vi "FPGA myRIOMain_v4.vi"() -> ()   [LabVIEW 2019]
doc: "Main FPGA VI\nUse the bitfile generated by this VI in the real-time code.\n\nFlip the channels for input and output"
uses:
  TypeDefs/AO mode TabCtrl.ctl
  TypeDefs/SamplingModeEnum.ctl
  <vilib>/rvi/Emulation/niFpgaGetClockAttributes.vi
  <vilib>/rvi/Emulation/niFpgaSctlEmulationGetInTimedLoop.vi
  <vilib>/rvi/Emulation/niFpgaEmulationReportErrorSimple.vi
  <vilib>/rvi/eio/common/nirviEmuTemplateMethod_errors.vi
  <vilib>/rvi/Emulation/niFpgaProcessEmulError.vi
  <vilib>/rvi/Emulation/niFpgaCriticalErrorInLSC.vi
  <vilib>/rvi/Emulation/niFpgaEmulationIsFPGAContextNoSignature.vi
  <vilib>/rvi/errors/niFpgaSetErrorForExecOnDevCompSimple.vi
  <vilib>/rvi/eio/common/nirviEmuReportErrorAndStop.vi
  <vilib>/rvi/DataTransferAndStorage/Container/Common/niFpgaContainerGetUniqueNameForEmu.vi
  <vilib>/rvi/FIFO/Fifo_Resource/nirvififoEmulationSetSize.vi
  <vilib>/rvi/FIFO/Fifo_Resource/nirviFifoEmulationQueueMgr.vi
  <instcachedir>/0/nirviFifoEmulationQueueMgr_E5CAEC123FF24DC58D834DCA3CDAA9B5.lvgen/nirviFifoEmulationQueueMgr_E5CAEC123FF24DC58D834DCA3CDAA9B5_003.vi
  <vilib>/Utility/error.llb/Clear Errors.vi
  <vilib>/rvi/FIFO/Fifo_Resource/nirvififoEmulationCreateLock.vi
  <vilib>/rvi/FIFO/Fifo_Resource/nirvififoEmulationObtainLock.vi
  <vilib>/rvi/FIFO/Fifo_Resource/nirvififoEmulationReleaseLock.vi
  <vilib>/rvi/occurrence/nirviWaitOnOccurrenceBase.vi
  <vilib>/rvi/errors/nirviReportUnexpectedCaseInternalError.vi
  <vilib>/rvi/errors/nirviReportUnexpectedCaseInternalError (U32).vi
  <vilib>/rvi/FIFO/Fifo_Resource/nirvififoEmulationDetermineInputValidOut.vi
  <vilib>/eio/EIONode/EIONode.xnode
  <vilib>/rvi/DataTransferAndStorage/Container/XNode/niFpgaContainer.xnode
  <vilib>/rvi/FIFO/Fifo_Resource/nirvififoEmulationRead.vi
  <vilib>/rvi/Analysis/measure/butterworth/XNode/niFpgaButterworthFilter.xnode
  <vilib>/rvi/FXPMathLib/FxpMul/XNode/nifxpmath_Multiplier.xnode
  <vilib>/rvi/FIFO/Fifo_Resource/nirvififoEmulationWrite.vi
  FPGA functions/FPGA functions.lvlib
  <vilib>/rvi/FXPMathLib/sim/FxpSim.dll
panel:
  in  "AI Process Time [ticks]":u32=120
  out "Sample Freq. \ntoo high?":bool
  out "Processing Loop time [ticks]":u32
  out "AI Process. Freq.\ntoo high?":bool
  in  "Scaled Butterworth Coeffs":i32[](array[numeric])=[-1036986264, 2110353124, 93741, -1058362983, 2131726043, 94691]
  in  "Sampling Mode":T1
  in  "Bit-resolution":i8=12
  in  "AO mode":T2
  in  "AO Out [V]":fxp<+/-,18,5> format="%#.6g"
  in  "AO enable?":bool
  out "AI In [V]":fxp<+/-,25,5> format="%#.6g"
  out "FPGA AO DMA\nOverflow?":bool
  out "Int. Output":i16
  out "Raw Int. Input":i16
  in  "Sample Time [ticks]":u32=120
  out "AO Loop time [ticks]":u32
  out "AI Loop time [ticks]":u32
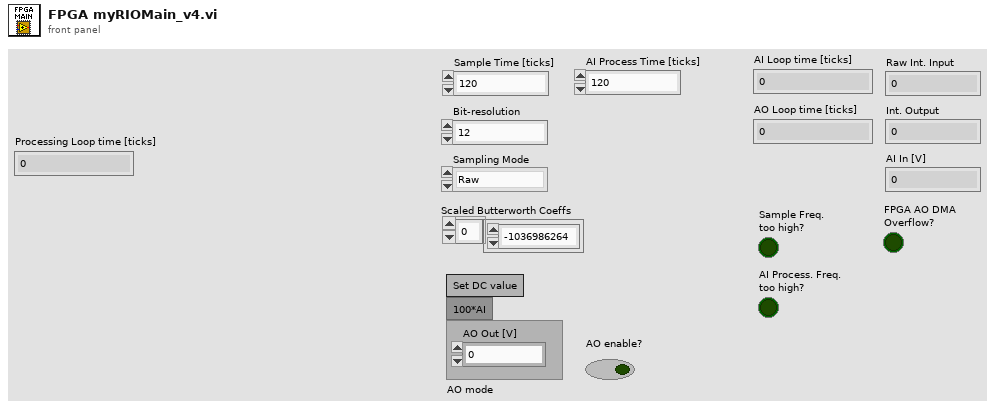
[diagram p1: front panel]
types:
  T1 = typedef "SamplingModeEnum.ctl" = enum16{"Raw", "LPF", "4 pt. Avg. + LPF"}
  T2 = typedef "AO mode TabCtrl.ctl" = enum32{"Set DC value", "100*AI"}
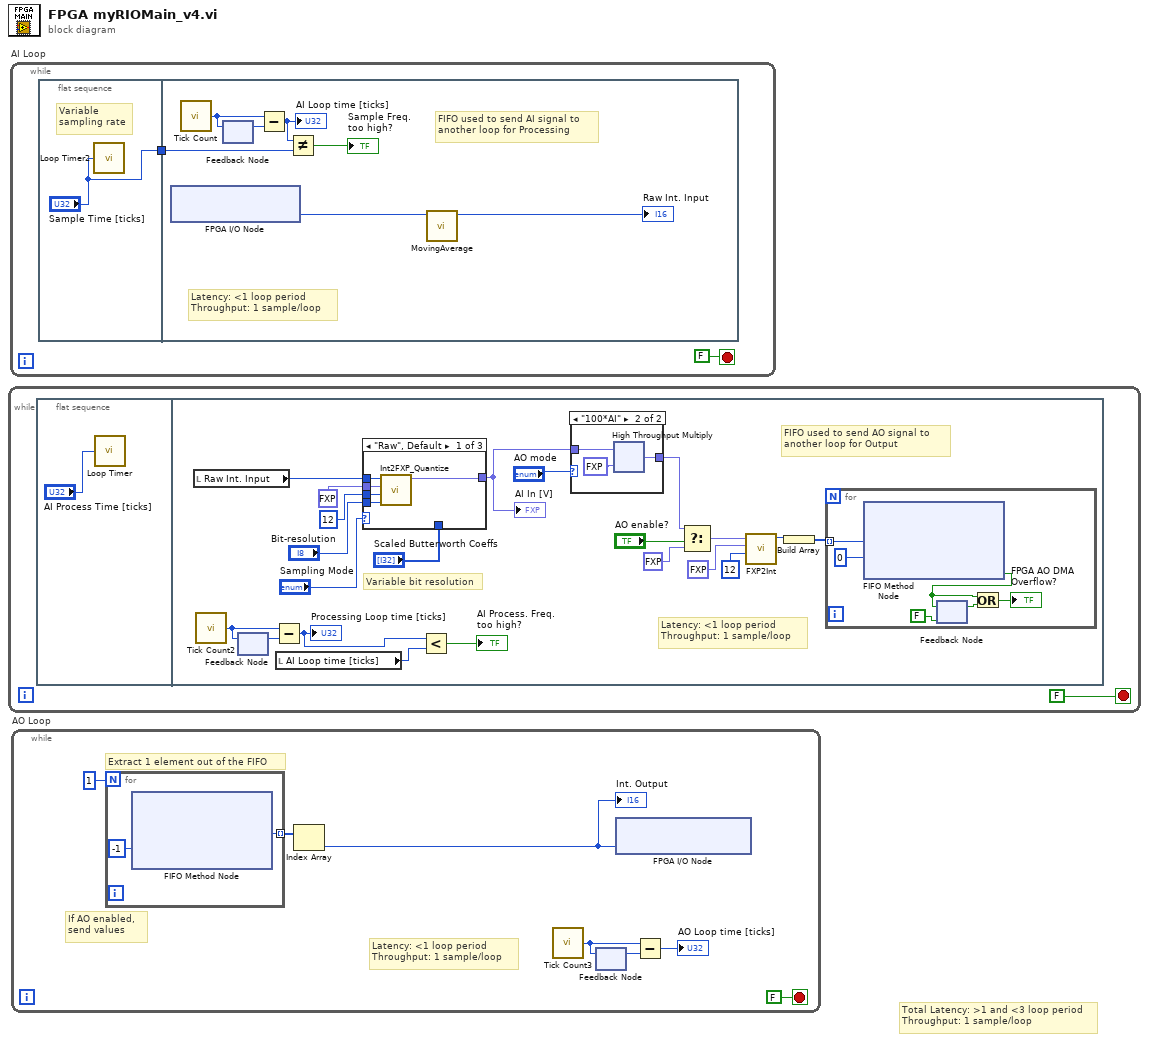
[diagram p0: block diagram]
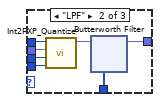
[diagram p2: hidden frame]
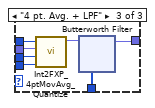
[diagram p3: hidden frame]
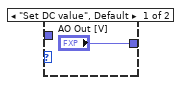
[diagram p4: hidden frame]
diagram:
  # "Total Latency: >1 and <3 loop period\nThroughput: 1 sample/loop"
  n1 = while {
    stop <- FALSE stop-if-true
    n2 = flat-sequence {
      frame #0 {
        n3 = call "Loop Timer"("Count(Ticks)"="AI Process Time [ticks]") -> ()  [unwired: 1 out]
      }
      frame #1 {
        # "Variable bit resolution"
        # "Latency: <1 loop period\nThroughput: 1 sample/loop"
        # "FIFO used to send AO signal to \nanother loop for Output"
        n4 = local read "Raw Int. Input"() -> (w6:i16)
        n5 = call "Tick Count2"() -> ("Tick Count(Ticks)"=w8:u32)
        n6 = feedback #1() -> (w7:u32)  [unwired: 1 in]
        n7 = feedback-in #1(w8) -> ()
        n8 = Subtract(x=w8, y=w7) -> (x-y=w4:u32)
        "Processing Loop time [ticks]" <- w4
        n9 = local read "AI Loop time [ticks]"() -> (w5:u32)
        n10 = case shown="\"Raw\", Default" "Sampling Mode" {
          tunnel: i8 12 ("Input Bit resolution") -> [w28 w32 w49]
          tunnel: fxp<+,8,4> 10.0 ("Multiplier") -> [w27 w33 w50]
          tunnel: "Bit-resolution" -> [w26 w31 w48]
          tunnel: "Scaled Butterworth Coeffs" -> [_ w34 w46]
          tunnel: [w25 w30 w45] -> w9
          tunnel: w6 -> [w24 w29 w44]
          frame "Raw", Default {
            n11 = call "Int2FXP_Quantize.vi"("Output Bit resolution"=w26, "Input Bit resolution"=w28, "Multiplier"=w27, "Input (Int)"=w24) -> ("Output (FXP)"=w25:fxp<+/-,25,5>)  [unwired: 7 in]
          }
          frame "LPF" {
            n12 = call "Int2FXP_Quantize.vi"("Output Bit resolution"=w31, "Input Bit resolution"=w32, "Multiplier"=w33, "Input (Int)"=w29) -> ("Output (FXP)"=w35:fxp<+/-,25,5>)  [unwired: 7 in]
            n13 = xnode "Butterworth Filter"("input data"=w35, "scaled coefficients"=w34) -> ("output data"=w30:fxp<+/-,25,5>)  [unwired: 1 in]
          }
          frame "4 pt. Avg. + LPF" {
            n14 = call "Int2FXP_4ptMovAvg_Quantize.vi"("Output Bit resolution"=w48, "Input Bit resolution"=w49, "Multiplier"=w50, "Input (Int)"=w44) -> ("Output (FXP)"=w47:fxp<+/-,25,5>)  [unwired: 7 in]
            n15 = xnode "Butterworth Filter"("input data"=w47, "scaled coefficients"=w46) -> ("output data"=w45:fxp<+/-,25,5>)  [unwired: 1 in]
          }
        }
        "AI In [V]" <- w9
        n16 = Less?(x=w4, y=w5) -> (x < y?=→"AI Process. Freq.\ntoo high?":bool)
        n17 = case shown="\"100*AI\"" "AO mode" {
          tunnel: ["AO Out [V]" w60] -> w16
          tunnel: w9 -> [_ w62]
          frame "Set DC value", Default {
          }
          frame "100*AI" {
            n18 = xnode ("High Throughput Multiply")("x"=w62, "y"=fxp<+,5,7> 100.0) -> ("x*y"=w60:fxp<+/-,18,5>)
          }
        }
        n19 = Select(t=w16, s="AO enable?", f=fxp<+/-,18,5> 0.0) -> (s? t:f=w17:fxp<+/-,18,5>)
        n20 = call "FXP2Int.vi"("Output Bit resolution"=i8 12 ("Bit resolution"), "Multiplier"=fxp<+,18,-1> 0.10000038146972656, "Input (FXP)"=w17) -> ("Output (Int)"=w23:i16)  [unwired: 8 in]
        n21 = Build Array(w23) -> (w18:i16[])
        n22 = for {
          tunnel: w18 -> [w65] mode=indexing
          n23 = xnode ("FIFO Method Node")("Element"=w65, "Timeout"=0) -> ("Timed Out?"=w63:bool)  [unwired: 1 in, 1 out]
          n24 = feedback-in #2(w63) -> ()
          n25 = feedback #2(FALSE ("Timed Out?")) -> (w67:bool)
          n26 = Or(x=w63, y=w67) -> (x .or. y?=→"FPGA AO DMA\nOverflow?":bool)
        }
      }
    }
  }
  n27 = while "AI Loop" {
    stop <- FALSE stop-if-true
    n28 = flat-sequence {
      tunnel: ["Sample Time [ticks]"] -> w69
      tunnel: w69 -> [w75]
      frame #0 {
        # "Variable\nsampling rate"
        n29 = call "Loop Timer2"("Count(Ticks)"="Sample Time [ticks]") -> ()  [unwired: 1 out]
      }
      frame #1 {
        # "FIFO used to send AI signal to \nanother loop for Processing"
        # "Latency: <1 loop period\nThroughput: 1 sample/loop"
        n30 = xnode "FPGA I/O Node"() -> ("ConnectorC/AI0"=w72:i16)  [unwired: 1 in, 1 out]
        n31 = call "Tick Count"() -> ("Tick Count(Ticks)"=w78:u32)
        n32 = feedback #3() -> (w77:u32)  [unwired: 1 in]
        n33 = feedback-in #3(w78) -> ()
        n34 = Subtract(x=w78, y=w77) -> (x-y=w76:u32)
        "AI Loop time [ticks]" <- w76
        n35 = Not Equal?(x=w76, y=w75) -> (x != y?=→"Sample Freq. \ntoo high?":bool)
        n36 = call "MovingAverage.vi"("Raw input"=w72) -> ("Avg. output"=→"Raw Int. Input":i16)  [unwired: 10 in]
      }
    }
  }
  n37 = while "AO Loop" {
    stop <- FALSE stop-if-true
    # "Latency: <1 loop period\nThroughput: 1 sample/loop"
    # "If AO enabled, \nsend values"
    # "Extract 1 element out of the FIFO"
    n38 = for {
      N: 1 -> [_]
      tunnel: [w87] -> w81 mode=indexing
      n39 = xnode ("FIFO Method Node")("Timeout"=-1) -> ("Element"=w87:i16)  [unwired: 1 in, 2 out]
    }
    n40 = Index Array(array=w81) -> (element=w79:i16)  [unwired: 1 in]
    "Int. Output" <- w79
    n41 = call "Tick Count3"() -> ("Tick Count(Ticks)"=w84:u32)
    n42 = feedback #4() -> (w83:u32)  [unwired: 1 in]
    n43 = feedback-in #4(w84) -> ()
    n44 = xnode "FPGA I/O Node"("ConnectorC/AO0"=w79) -> ()  [unwired: 1 in, 1 out]
    n45 = Subtract(x=w84, y=w83) -> (x-y=→"AO Loop time [ticks]":u32)
  }
